vi "Configure PRACH Sequence Index.vi"(7 "Sequence Index (0)":i32, 8 "error in (no error)":errorcluster, 9 "Sequence Index Auto (On)":bool=TRUE, 10 "Instance (1)":T1=1, 11 "VISA resource name":refnum<visa-resource-name>) -> (0 "error out":errorcluster, 3 "VISA resource name out":refnum<visa-resource-name>)   [LabVIEW 2020, in "Rohde&Schwarz CMWXP NR FR1 Measurement.lvlib"]
doc: "Enables or disables automatic detection of the sequence index. Specifies the sequence index, i.e. which of the 64 preamble sequences of the cell is used by the UE, if automatic detection is disabled.\n\nAttributes:\nRSCMWXPNRFR1M_ATTR_PRACH_SEQUENCE_INDEX_ENABLED\nRSCMWXPNRFR1M_ATTR_PRACH_SEQUENCE_INDEX\n\nRemote-control commands:\nCONFigure:NRSub:MEAS<i>:PRACh:SINDex:AUTO\nCONFigure:NRSub:MEAS<i>:PRACh:SINDex"
uses:
  <instrlib>/Rohde&Schwarz CMWXP NR FR1 Measurement/Rohde&Schwarz CMWXP NR FR1 Measurement.lvlib
  <instrlib>/Rohde&Schwarz CMWXP NR FR1 Measurement/Private/_Instance.ctl
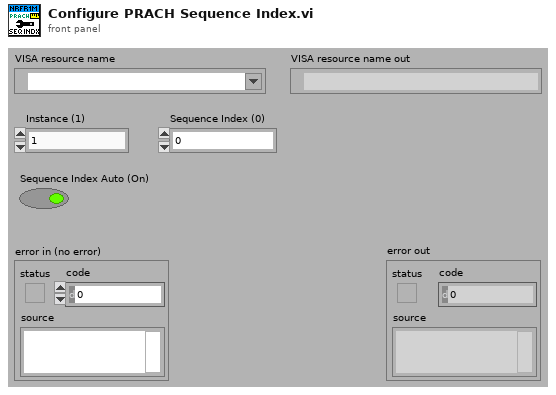
[diagram p1: front panel]
types:
  T1 = typedef "Rohde&Schwarz CMWXP NR FR1 Measurement.lvlib/_Instance.ctl" = i32
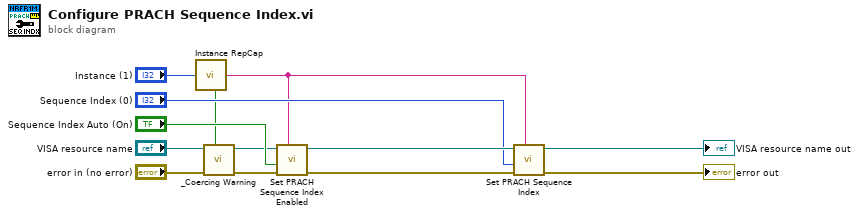
[diagram p0: block diagram]
diagram:
  n1 = call <instrlib>:"Instance RepCap.vi"("Instance In"="Instance (1)") -> ("In Range?"=w2:bool, "RepCap Identifier Out"=w1:string)  [unwired: 1 in]
  n2 = call <instrlib>:"_Coercing Warning.vi"("In Range?"=w2, "error in (no error)"="error in (no error)", "VISA resource name"="VISA resource name") -> ("error out"=w5:errorcluster, "VISA resource name out"=w4:refnum<visa-resource-name>)  [unwired: 7 in]
  n3 = call "Set PRACH Sequence Index Enabled"("Repeated Capabilities"=w1, "error in (no error)"=w5, "PRACH Sequence Index Enabled (OFF)"="Sequence Index Auto (On)", "instrument handle"=w4) -> ("error out"=w9:errorcluster, "instrument handle out"=w10:refnum<visa-resource-name>)  [unwired: 6 in]
  n4 = call "Set PRACH Sequence Index"("Repeated Capabilities"=w1, "error in (no error)"=w9, "PRACH Sequence Index (0)"="Sequence Index (0)", "instrument handle"=w10) -> ("error out"=→"error out":errorcluster, "instrument handle out"=→"VISA resource name out":refnum<visa-resource-name>)  [unwired: 6 in]
